vi "LS372 _Set_ver1.0.vi"(0 "AutoRange?":bool, 2 "error in":errorcluster, 4 "Voltage":u16(ring) items=["2.00 uV"=1, "6.32 uV"=2, "20.0 uV"=3, "63.2 uV"=4, "200 uV"=5, "632 uV"=6, "2.0 mV"=7, "6.32 mV"=8], 5 "Range (Ohms)":u16(ring) items=["2.0 m"=1, "6.32 m"=2, "20.0 m"=3, "63.2 m"=4, "200 m"=5, "632 m"=6, "2.00"=7, "6.32"=8, "20.0"=9, "63.2"=10, "200"=11, "632"=12, "2.00 k"=13, "6.32 k"=14, "20.0 k"=15, "63.2 k"=16, "200 k"=17, "632 k"=18, "2.00 M"=19, "6.32 M"=20, "20.0 M"=21, "63.2 M"=22], 6 "Current":u16(ring) items=["1.00 pA"=1, "3.16 pA"=2, "10.0 pA"=3, "31.6 pA"=4, "100 pA"=5, "316 pA"=6, "1.00 nA"=7, "3.16 nA"=8, "10 nA"=9, "31.6 nA"=10, "100 nA"=11, "316 nA"=12, "1.00 uA"=13, "3.16 uA"=14, "10.0 uA"=15, "31.6 uA"=16, "100 uA"=17, "316 uA"=18, "1.00 mA"=19, "3.16 mA"=20, "10.0 mA"=21, "31.6 mA"=22], 7 "Excitation mode":u16(ring) items=["Voltage Excitation", "Current Excitation"], 8 "GPIB ADR":u16) -> (1 "error out":errorcluster, 3 "dump GPIB ADR":u16)   [LabVIEW 2012]
panel:
  in  "Unit":u16(ring)=2 items=["Kelvin"=1, "Ohms"=2]
  in  "Current source shunted?":bool
  in  "Input  Channel":u16(ring)=1 items=["All Channels", "Input 1", "Input 2", "Input 3", "Input 4", "Input 5", "Input 6", "Input 7", "Input 8"]
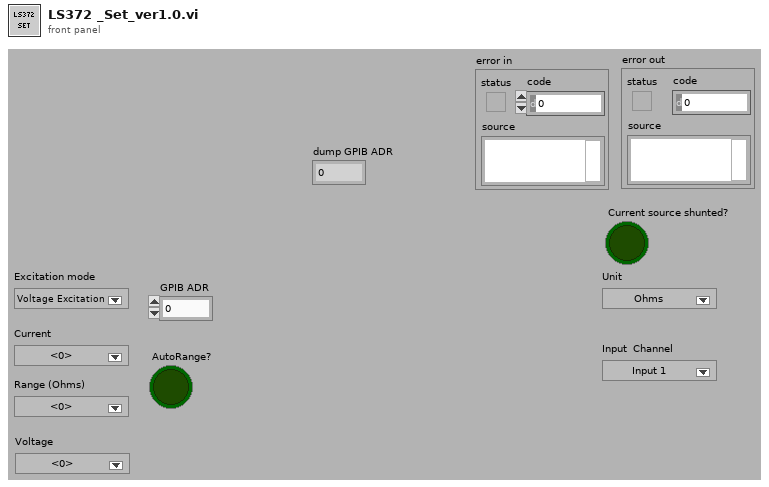
[diagram p1: front panel]
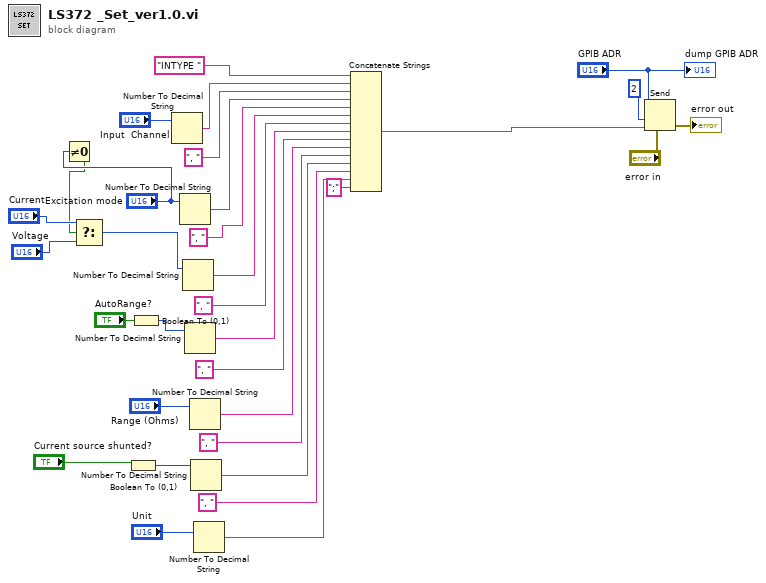
[diagram p0: block diagram]
diagram:
  n1 = Not Equal To 0?(x="Excitation mode") -> (x != 0?=w3:bool)
  n2 = Select(t="Current", s=w3, f="Voltage") -> (s? t:f=w2:u16)
  n3 = Boolean To (0,1)(Boolean="Current source shunted?") -> (0, 1=w16:i16)
  n4 = Boolean To (0,1)(Boolean="AutoRange?") -> (0, 1=w21:i16)
  n5 = Number To Decimal String(number="Input  Channel") -> (decimal integer string=w30:string)  [unwired: 1 in]
  n6 = Number To Decimal String(number="Excitation mode") -> (decimal integer string=w28:string)  [unwired: 1 in]
  n7 = Number To Decimal String(number=w2) -> (decimal integer string=w26:string)  [unwired: 1 in]
  n8 = Number To Decimal String(number=w21) -> (decimal integer string=w23:string)  [unwired: 1 in]
  n9 = Number To Decimal String(number="Range (Ohms)") -> (decimal integer string=w19:string)  [unwired: 1 in]
  n10 = Number To Decimal String(number=w16) -> (decimal integer string=w15:string)  [unwired: 1 in]
  n11 = Number To Decimal String(number="Unit") -> (decimal integer string=w12:string)  [unwired: 1 in]
  n12 = Concatenate Strings("INTYPE " ("format string"), w30, ", " ("format string"), w28, ", " ("format string"), w26, ", " ("format string"), w23, ", " ("format string"), w19, ", " ("format string"), w15, ", " ("format string"), w12, ";" ("string")) -> (w7:string)
  n13 = Send(2:"GPIB ADR", 3:i16 2 ("mode"), 4:"error in", 5:w7) -> (8:→"error out":errorcluster)  [unwired: 1 in, 2 out]
  "dump GPIB ADR" <- "GPIB ADR"
